vi "counter 1 with semaphore.vi"() -> ()   [LabVIEW 2010]
panel:
  out "카운트 1":i32
  out "진행 중 합계":i32
  in  "정지":bool
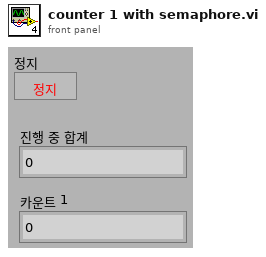
[diagram p1: front panel]
types:
  T1 = typedef "Semaphore RefNum" = refnum<k1>
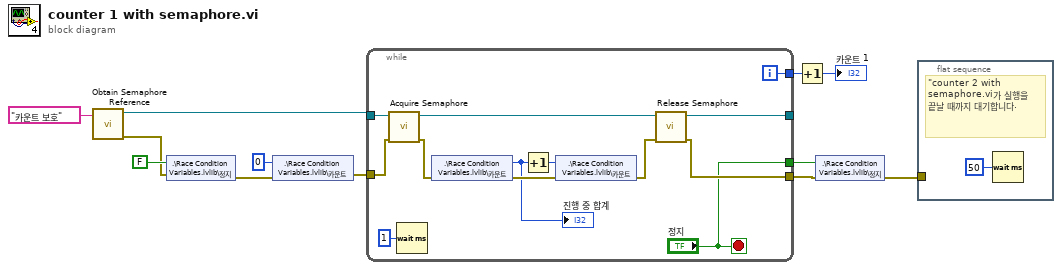
[diagram p0: block diagram]
diagram:
  n1 = call <vilib>:"Obtain Semaphore Reference.vi"("name (unnamed)"="카운트 보호") -> ("error out"=w3:errorcluster, "semaphore"=w2:T1)  [unwired: 4 in, 1 out]
  n2 = shared-variable ".\\Race Condition Variables.lvlib\\정지"(FALSE ("stop"), error in=w3) -> (error out=w6:errorcluster)
  n3 = shared-variable ".\\Race Condition Variables.lvlib\\카운트"(0 ("counter"), error in=w6) -> (error out=w12:errorcluster)
  n4 = while {
    tunnel: [w24] -> w11
    tunnel: w12 -> [w19]
    tunnel: w2 -> [w20]
    tunnel: [w15] -> _
    tunnel: [w14] -> w8
    tunnel: ["정지"] -> w7
    i -> [w24]
    stop <- "정지" stop-if-true
    n5 = call <vilib>:"Acquire Semaphore.vi"("error in (no error)"=w19, "semaphore"=w20) -> ("error out"=w18:errorcluster, "semaphore out"=w16:T1)  [unwired: 3 in, 1 out]
    n6 = Wait (ms)(milliseconds to wait=u32 1) -> ()  [unwired: 1 out]
    n7 = shared-variable ".\\Race Condition Variables.lvlib\\카운트"(error in=w18) -> (w21:i32, error out=w25:errorcluster)
    "진행 중 합계" <- w21
    n8 = Increment(x=w21) -> (x+1=w22:i32)
    n9 = shared-variable ".\\Race Condition Variables.lvlib\\카운트"(w22, error in=w25) -> (error out=w17:errorcluster)
    n10 = call <vilib>:"Release Semaphore.vi"("error in (no error)"=w17, "semaphore"=w16) -> ("error out"=w14:errorcluster, "semaphore out"=w15:T1)  [unwired: 4 in]
  }
  n11 = Increment(x=w11) -> (x+1=→"카운트 1":i32)
  n12 = shared-variable ".\\Race Condition Variables.lvlib\\정지"(w7, error in=w8) -> (error out=w4:errorcluster)
  n13 = flat-sequence {
    tunnel: w4 -> [_]
    frame #0 {
      # "\"counter 2 with semaphore.vi가 실행을 끝날 때까지 대기합니다."
      n14 = Wait (ms)(milliseconds to wait=u32 50) -> ()  [unwired: 1 out]
    }
  }
